vi "Stepper Control.vi"() -> ()   [LabVIEW 2018]
uses:
  <vilib>/LabVIEW Interface for Arduino/Type Defs/Board Type.ctl
  <vilib>/LabVIEW Interface for Arduino/Type Defs/Connection Type.ctl
  <vilib>/LabVIEW Interface for Arduino/LabVIEW Interface for Arduino.lvlib
panel:
  out "error out":errorcluster
  out "Iteration":i32
  in  "Baud Rate (115200)":u32=115200
  out "Step Angle":dbl
  in  "Step Size":i16
  out "Steps Remaining?":bool
  in  "Set Acceleration (0 to disable)":i16
  in  "Set Speed (Steps per Second)":i16=100
  in  "Steps for one rotation":i16
  in  "Control Method":u8(ring)=1 items=["2 Wire (Pulse & Direction)"=1, "2 Wire"=2, "4 Wire"=4, "EasyDriver"=6, "AF Motor Shield (Stepper 1 & 2 Only)"=5]
  in  "Stepper Pins":u8[](array[numeric])=[2, 3]
  in  "Stepper #":u8
  in  "error in":errorcluster
  in  "Board Type (Uno)":T1
  in  "VISA resource":refnum<visa-resource-name>
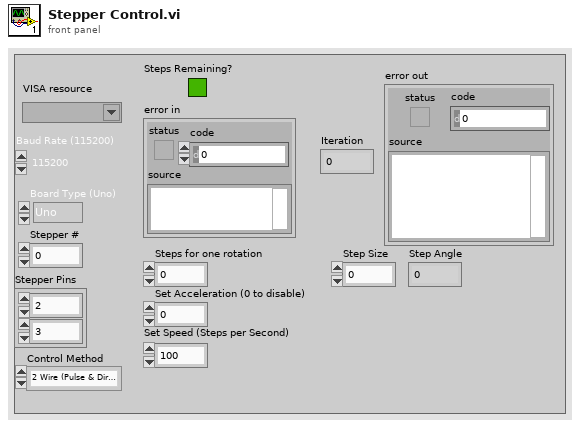
[diagram p1: front panel]
types:
  T1 = typedef "LabVIEW Interface for Arduino.lvlib/Board Type.ctl" = enum16{"Uno", "Dimuelanove w/Atmega 328", "Mega 2560"}
  T2 = typedef "LabVIEW Interface for Arduino.lvlib/Connection Type.ctl" = enum8{"USB / Serial", "XBEE", "BlueSmirf (Bluetooth)"}
  T3 = typedef "LabVIEW Interface for Arduino.lvlib/Arduino Resource.ctl" = cluster{"VISA resource":refnum<visa-resource-name>, "Board Type":T1, "Connection Type":enum8{"USB / Serial"}, "Bytes Per Packet (15)":u8}
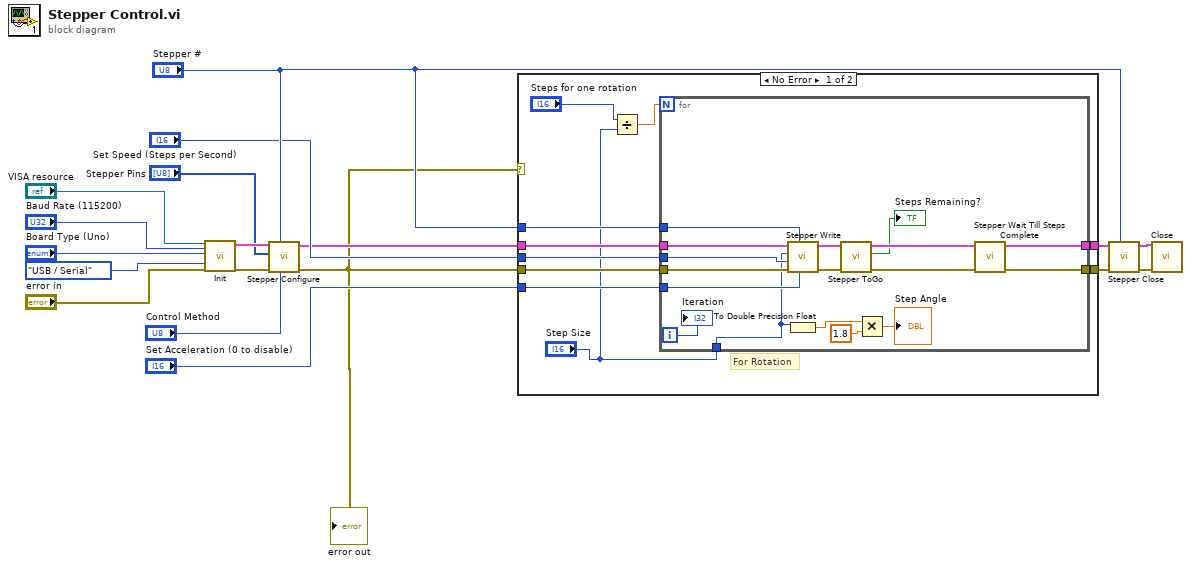
[diagram p0: block diagram]
diagram:
  n1 = call <vilib>:"Init.vi"("VISA resource"="VISA resource", "Baud Rate (115200)"="Baud Rate (115200)", "Board Type (Uno)"="Board Type (Uno)", "Connection Type (USB/Serial)"=Connection_Type."USB / Serial", "error in"="error in") -> ("Arduino Resource"=w15:T3, "error out"=w14:errorcluster)  [unwired: 13 in]
  n2 = call <vilib>:"Stepper Configure.vi"("Control Method"="Control Method", "Stepper #"="Stepper #", "error in"=w14, "Stepper Pins"="Stepper Pins", "Arduino Resource"=w15) -> ("error out"=w1:errorcluster, "Arduino Resource Out"=w3:T3)  [unwired: 5 in]
  "error out" <- w1
  n3 = case shown="No Error" w1 {
    tunnel: [w28 w46] -> w8
    tunnel: [w27 w47] -> w7
    tunnel: "Set Acceleration (0 to disable)" -> [w26 _]
    tunnel: "Stepper #" -> [w25 _]
    tunnel: w1 -> [w24 w46]
    tunnel: "Set Speed (Steps per Second)" -> [w23 _]
    tunnel: w3 -> [w22 w47]
    frame No Error {
      # "For Rotation"
      n4 = Divide(x="Steps for one rotation", y="Step Size") -> (x/y=w20:dbl)
      n5 = for {
        N: w20 -> [_]
        tunnel: [w42] -> w28
        tunnel: [w41] -> w27
        tunnel: w26 -> [w40]
        tunnel: w25 -> [w39]
        tunnel: w24 -> [w38]
        tunnel: w23 -> [w37]
        tunnel: w22 -> [w36]
        tunnel: "Step Size" -> [w29]
        i -> [w30]
        n6 = call <vilib>:"Stepper Write.vi"("Set Acceleration (0 to disable)"=w40, "Stepper #"=w39, "error in"=w38, "Set Speed (Steps per Second)"=w37, "# of Steps to Move"=w29, "Arduino Resource"=w36) -> ("error out"=w35:errorcluster, "Arduino Resource Out"=w34:T3)  [unwired: 4 in]
        n7 = To Double Precision Float(number=w29) -> (double precision float=w32:dbl)
        n8 = call <vilib>:"Stepper ToGo.vi"("error in"=w35, "Arduino Resource"=w34) -> ("error out"=w45:errorcluster, "Steps Remaining?"=→"Steps Remaining?":bool, "Arduino Resource Out"=w44:T3)  [unwired: 6 in, 1 out]
        n9 = Multiply(x=w32, y=1.8) -> (x*y=→"Step Angle":dbl)
        n10 = call <vilib>:"Stepper Wait Till Steps Complete.vi"("error in"=w45, "Arduino Resource In"=w44) -> ("error out"=w42:errorcluster, "Arduino Resource Out"=w41:T3)  [unwired: 8 in]
        "Iteration" <- w30
      }
    }
    frame Error {
    }
  }
  n11 = call <vilib>:"Stepper Close.vi"("Stepper #"="Stepper #", "error in"=w8, "Arduino Resource"=w7) -> ("error out"=w9:errorcluster, "Arduino Resource Out"=w10:T3)  [unwired: 7 in]
  n12 = call <vilib>:"Close.vi"("Arduino Resource"=w10, "error in"=w9) -> ()  [unwired: 13 in, 1 out]
